vi "Stopping.vi"(6 "Teller":refnum<class "Teller.lvclass">, 8 "Error in":errorcluster, 11 "Stopping jettl Msg in":refnum<class "Stopping jettl Msg.lvclass">) -> (0 "Error out":errorcluster, 3 "Stopping jettl Msg out":refnum<class "Stopping jettl Msg.lvclass">)   [LabVIEW 2020, in "jettl.lvlib" / "Stopping jettl Msg.lvlib" / "Stopping jettl Msg.lvclass"]
doc: "jettl 6.12.1.94\nNathan Davis - Nathan Davis\nCopyright (c) 2026, Nathan Davis\nMIT"
uses:
  Stopping jettl Msg.lvclass
  Teller/Teller.lvclass
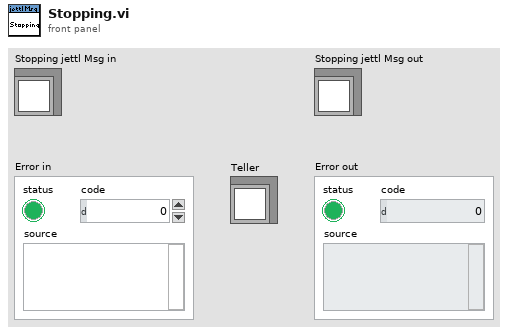
[diagram p1: front panel]
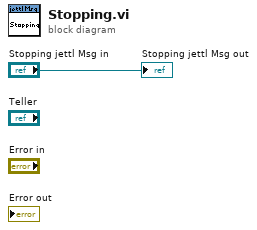
[diagram p0: block diagram]
diagram:
  "Stopping jettl Msg out" <- "Stopping jettl Msg in"
